vi "Car_Wash.vi"() -> ()   [LabVIEW 2021]
doc: "This is the car wash vi which simulates the car washing machine."
uses:
  Control/Queue_Operation_Select.ctl
  Control/Car_Wash_Data.ctl
  Control/Stage_Data.ctl
  Control/Timer_Operation_Select.ctl
  Control/Car_Wash_Indicators.ctl
  Control/INI_Operation_Select.ctl
  Control/Purchase_Selection.ctl
  Control/Car_Wash_Simulation_Switches.ctl
panel:
  out "Time":dbl format="%#_3g"
  out "Car_Wash_Indicators":T1 caption="Car Wash Indicators"
  in  "Stop":bool
  in  "Car_Wash_Simulation_Switches":T2 caption="Car Wash Simulation Switches"
  in  "Purchase_Selection":T3 caption="Purchase Selection"
  out "Error_Out":errorcluster
  in  "Error_In":errorcluster
  # "Sec"
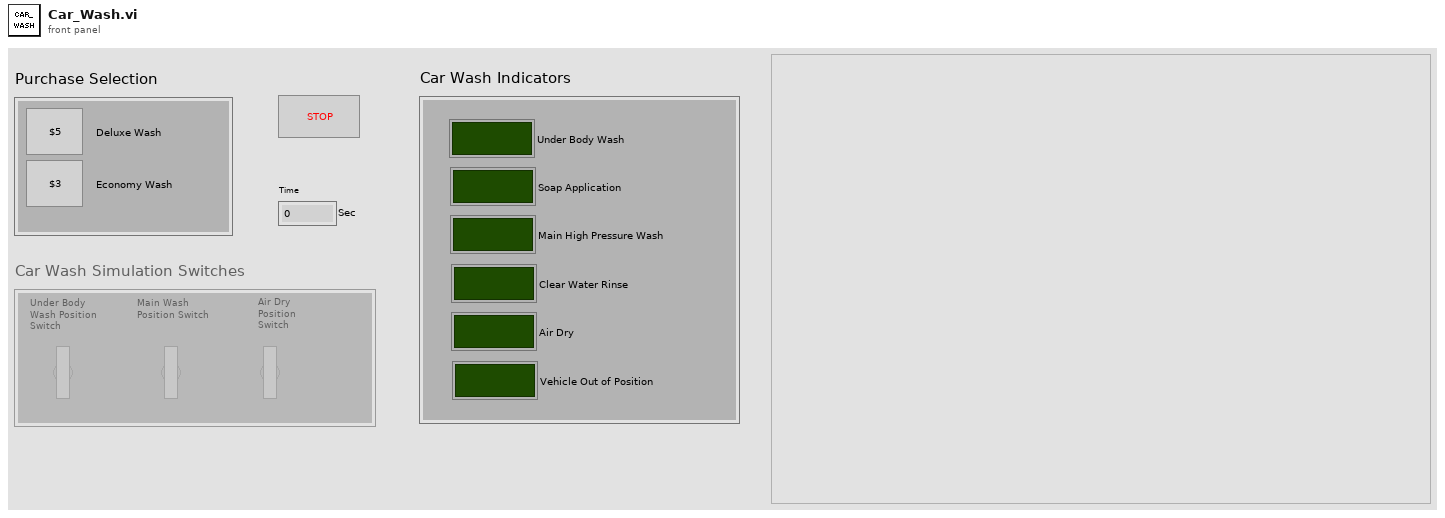
[diagram p1: front panel]
types:
  T1 = typedef "Car_Wash_Indicators.ctl" = cluster{"Under_Body_Wash":bool, "Soap_Application":bool, "Main_High_Pressure_Wash":bool, "Clear_Water_Rinse":bool, "Air_Dry":bool, "Vehicle_Out_of_Position":bool}
  T2 = typedef "Car_Wash_Simulation_Switches.ctl" = cluster{"Under_Body_Wash":bool, "Main_Wash":bool, "Dry_Wash":bool}
  T3 = typedef "Purchase_Selection.ctl" = cluster{"Deluxe_Wash":bool, "Economy_Wash":bool}
  T4 = typedef "Queue_Operation_Select.ctl" = enum16{"Obtain_Queue", "Enqueue", "Enqueue_N", "Enqueue_at_First", "Dequeue", "Flush_Queue", "Release_Queue"}
  T5 = typedef "Timer_Operation_Select.ctl" = enum16{"Start_Timer", "Pause_Timer", "Time_Out?", "Stop_Timer"}
  T6 = typedef "Car_Wash_Data.ctl" = cluster{"Car_Wash_Indicator_F":bool[], "Vehicle_Out_of_Position_F":bool, "Stage_1_Process_Data":T7[], "Stage_2_Process_Data":T7[], "Stage_3_Process_Data":T7[], "Stage_1_Process":i32, "Stage_2_Process":i32, "Stage_3_Process":i32, "Stage_1_Process_Started?":bool, "Stage_2_Process_Started?":bool, "Stage_3_Process_Started?":bool, "Current_Process_Stage":i32, "Enable_Control_Reference":refnum<vi>, "Disable_Control_Reference":refnum<vi>, "Car_Wash_Indicators":T1, "Latest_Car_Wash_Switch_Change":bool[], "Time":dbl}
  T7 = typedef "Stage_Data.ctl" = cluster{"Stage":i32, "Do?":bool, "Time_Required":i32}
  T8 = typedef "INI_Operation_Select.ctl" = enum16{"Read", "Write"}
  T9 = enum8{"Enabled", "Disabled", "Disabled and Grayed Out"}
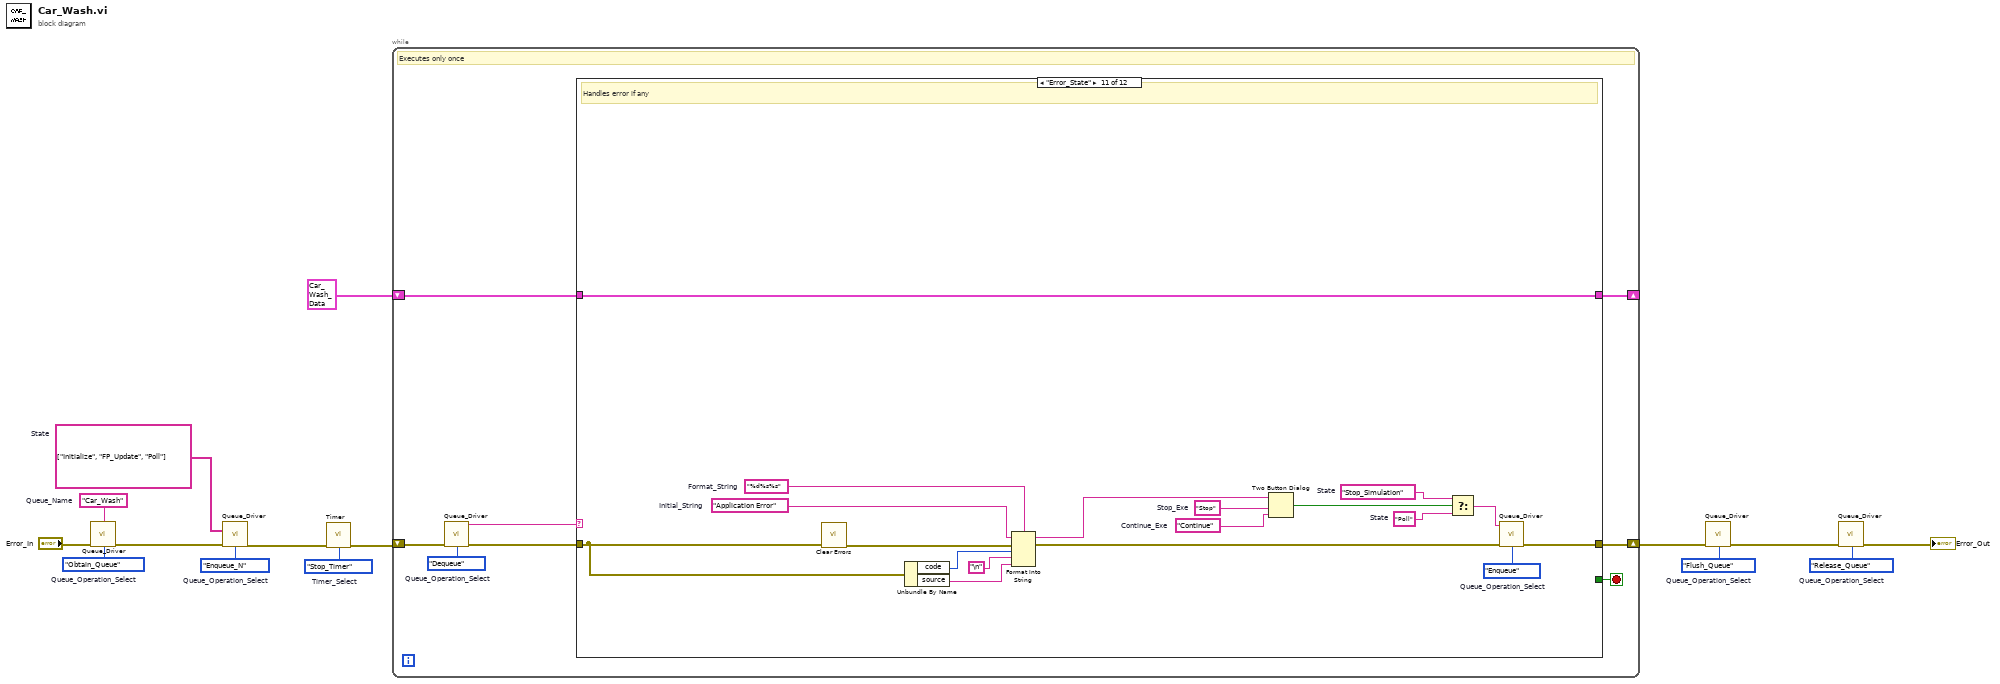
[diagram p0: block diagram]
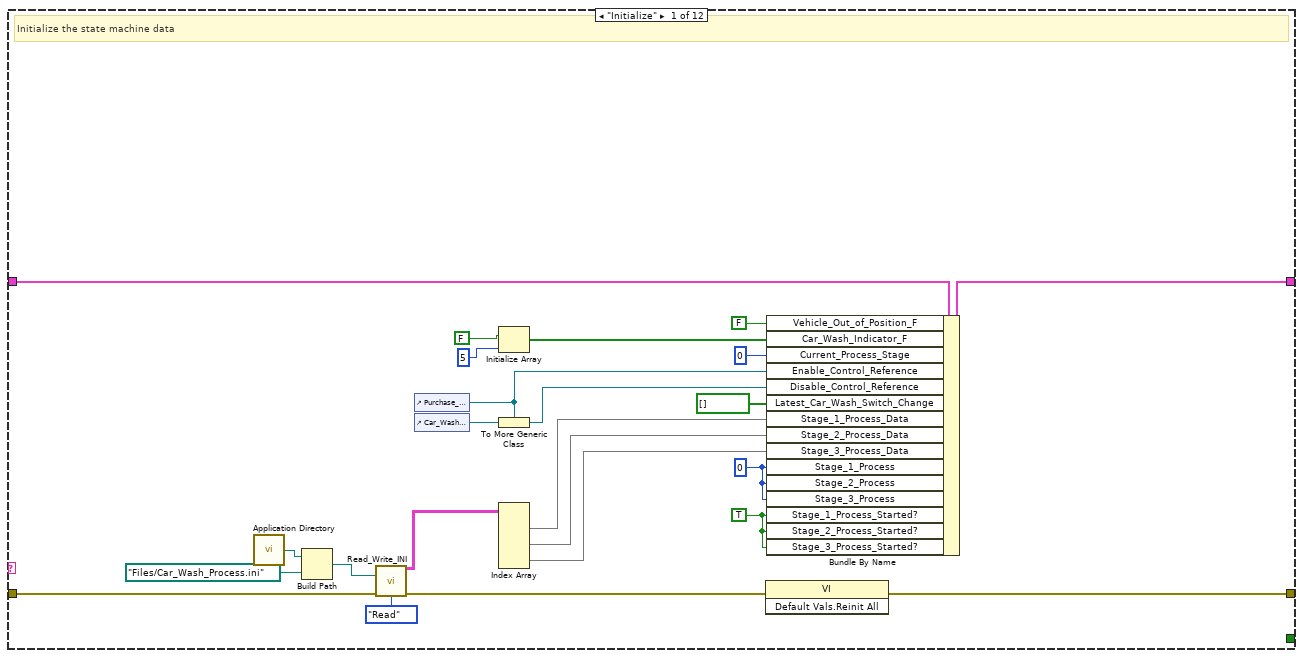
[diagram p2: hidden frame]
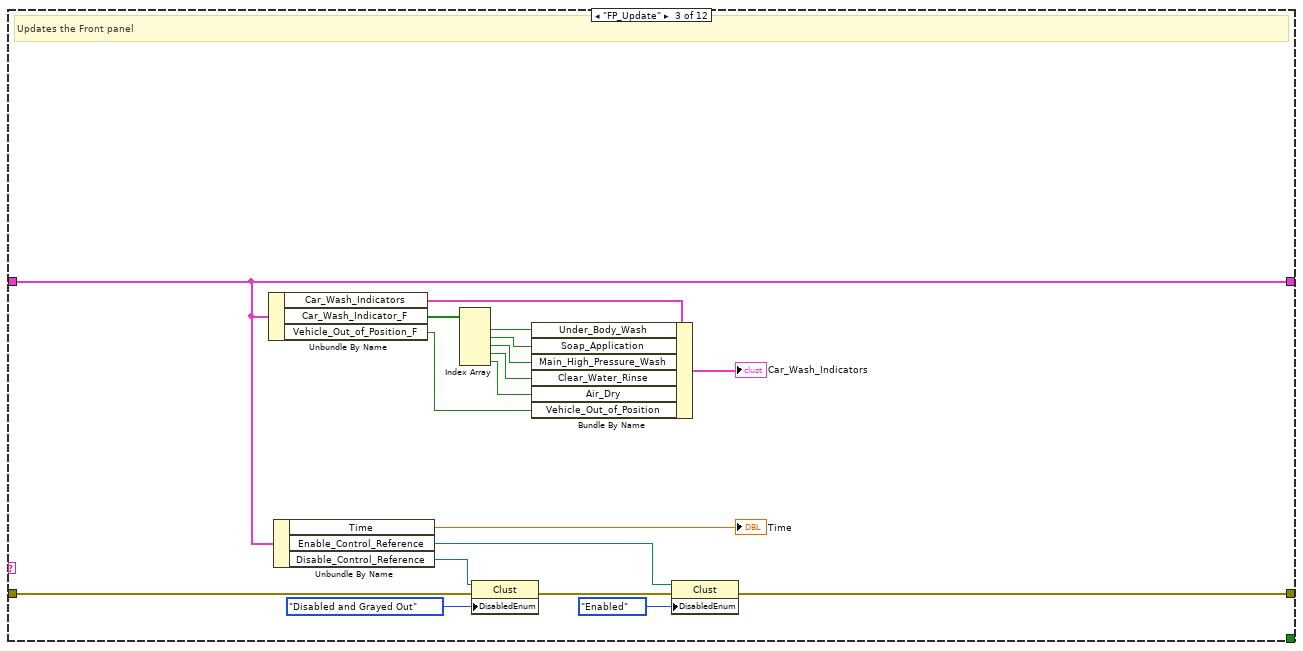
[diagram p4: hidden frame]
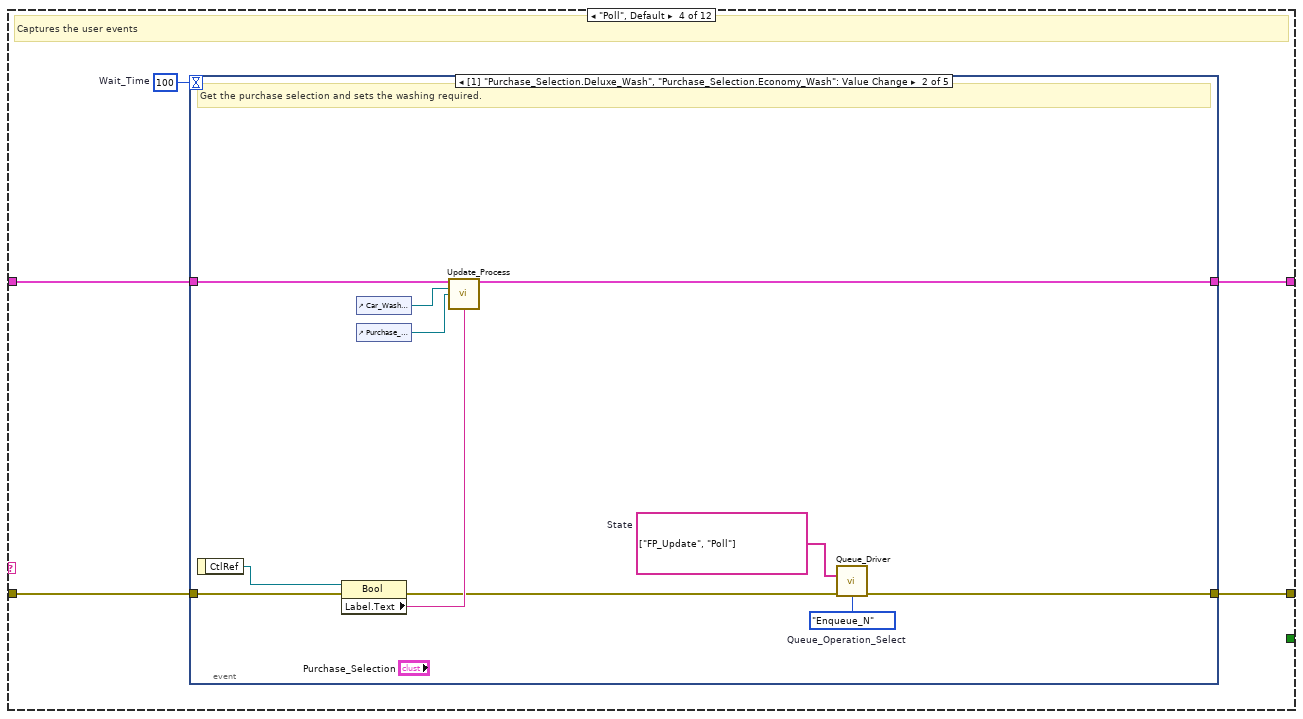
[diagram p5: hidden frame]
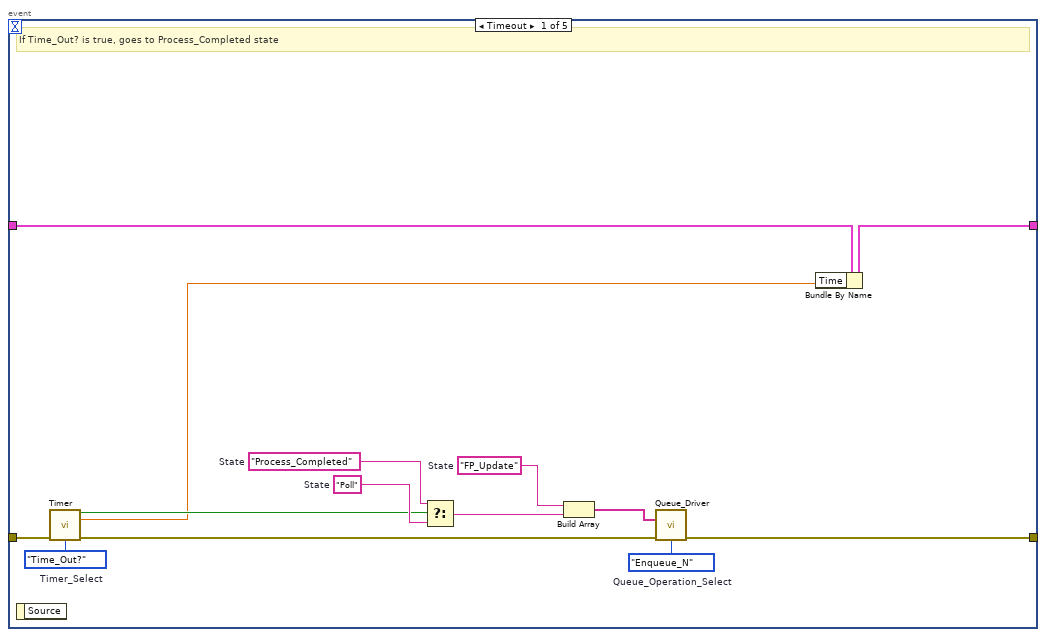
[diagram p6: hidden frame]
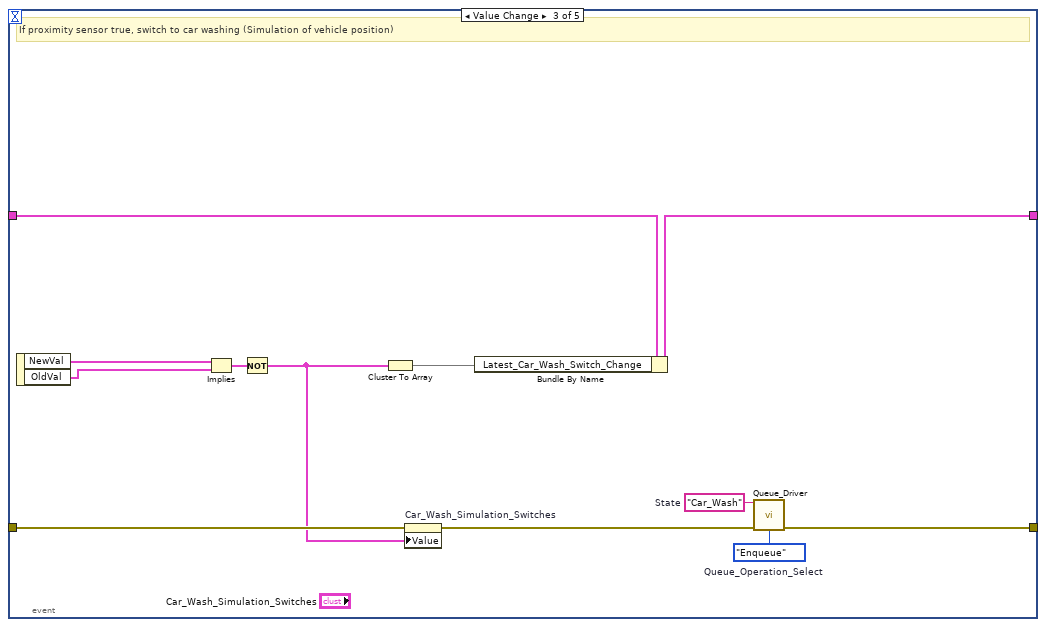
[diagram p7: hidden frame]
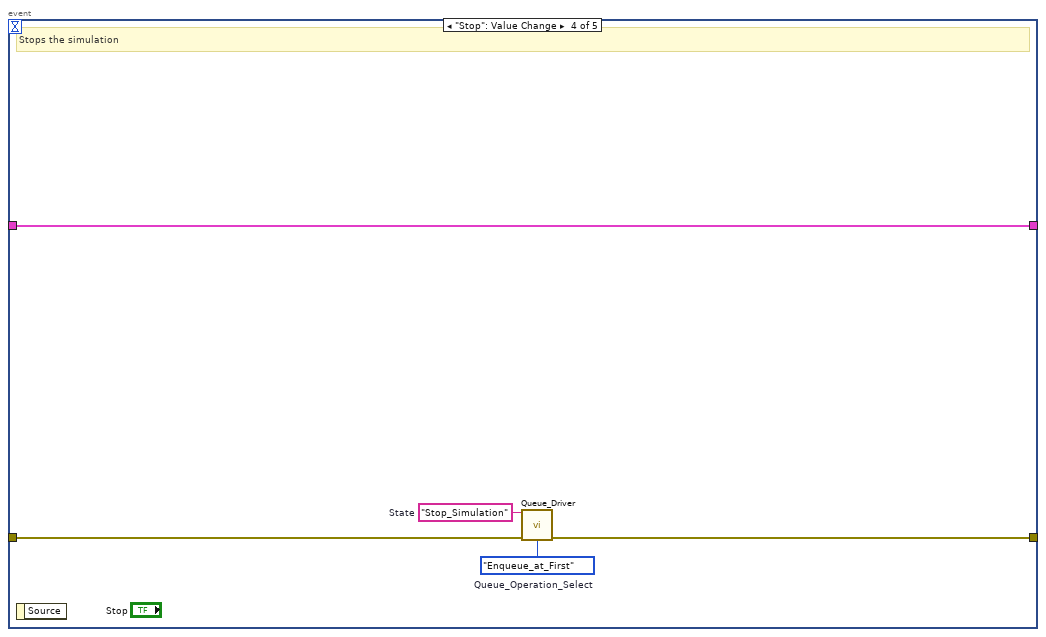
[diagram p8: hidden frame]
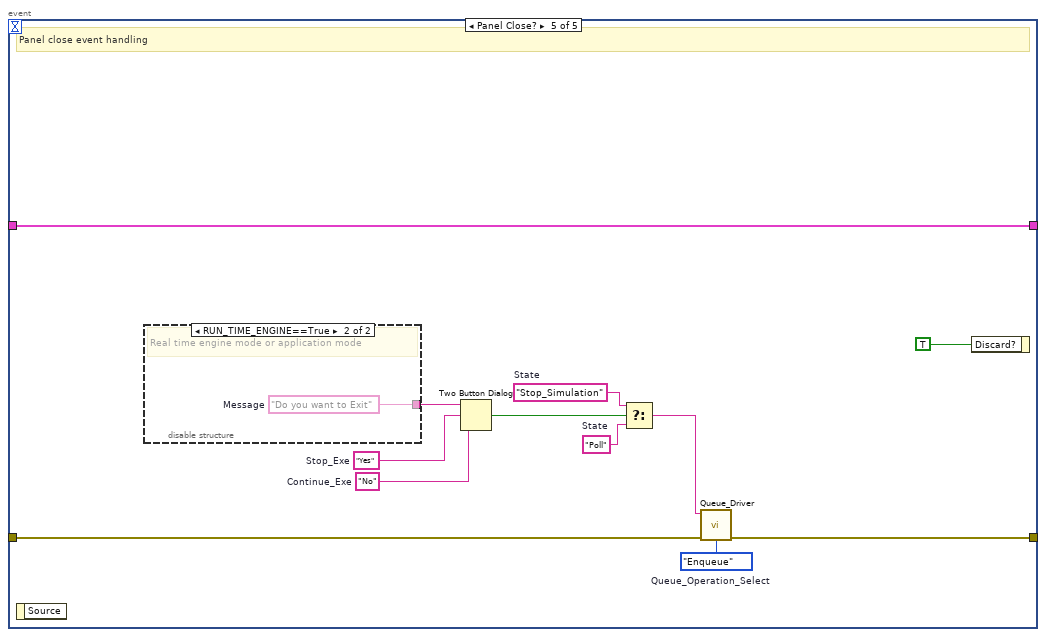
[diagram p9: hidden frame]
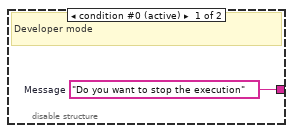
[diagram p10: hidden frame]
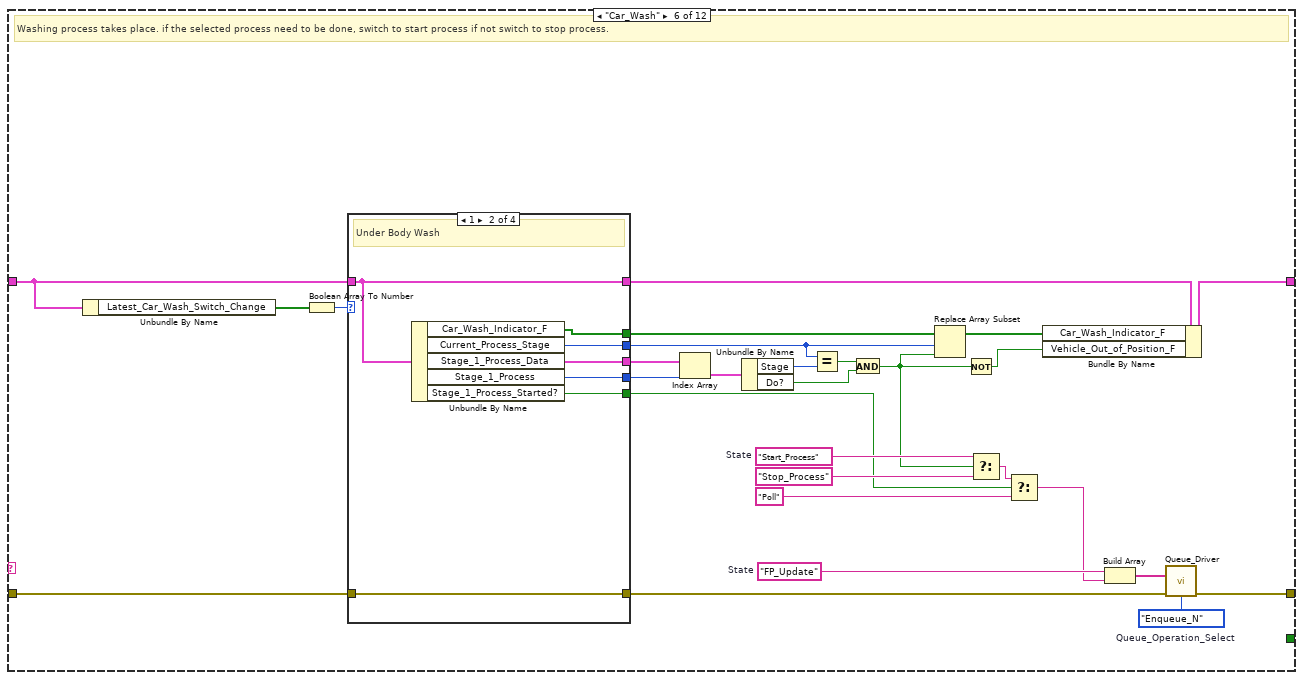
[diagram p12: hidden frame]
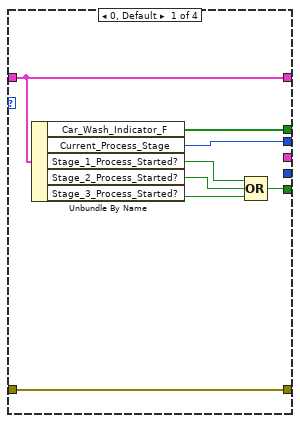
[diagram p13: hidden frame]
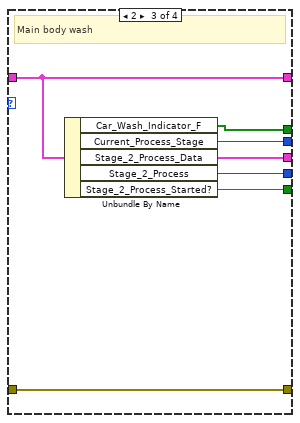
[diagram p14: hidden frame]
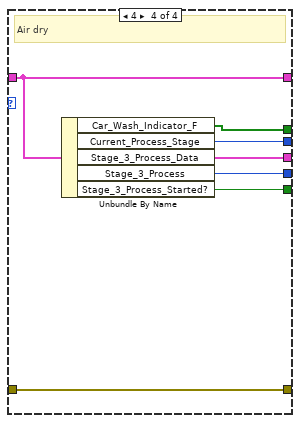
[diagram p15: hidden frame]
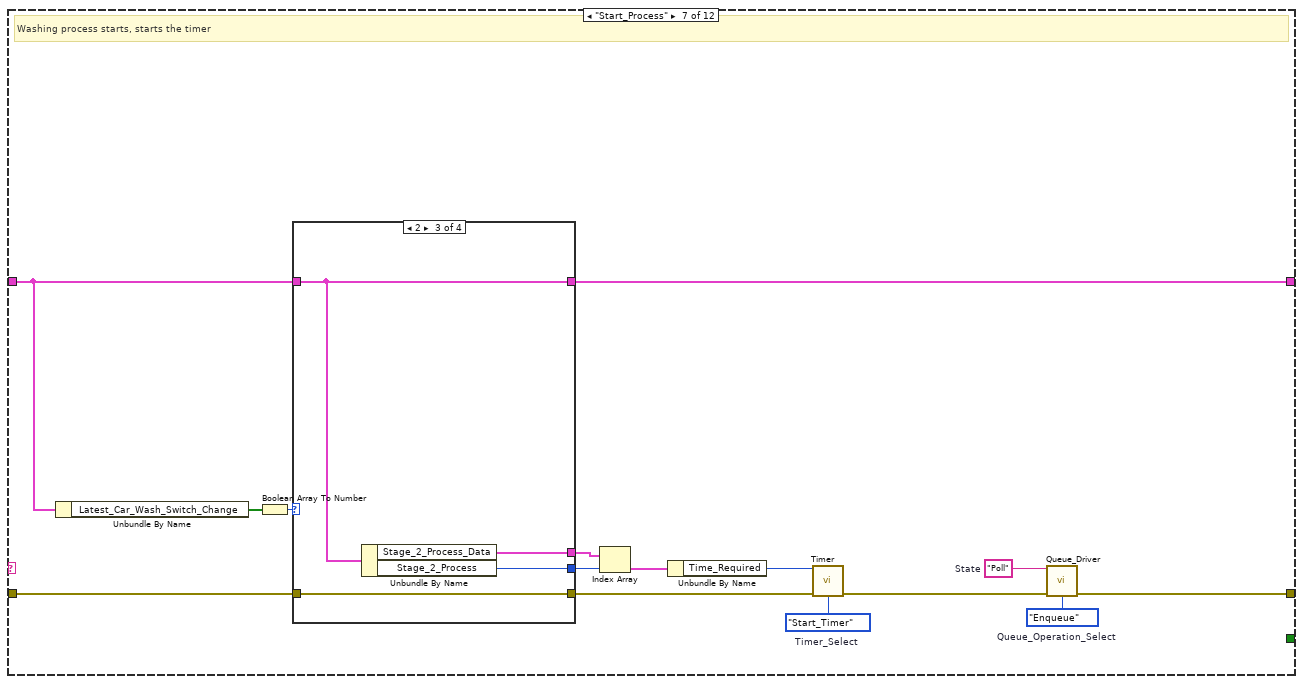
[diagram p16: hidden frame]
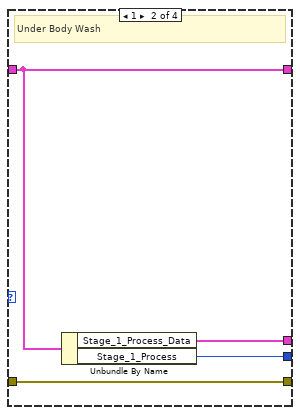
[diagram p18: hidden frame]
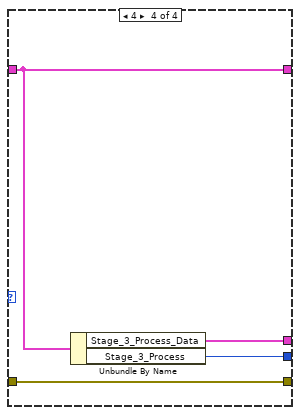
[diagram p19: hidden frame]
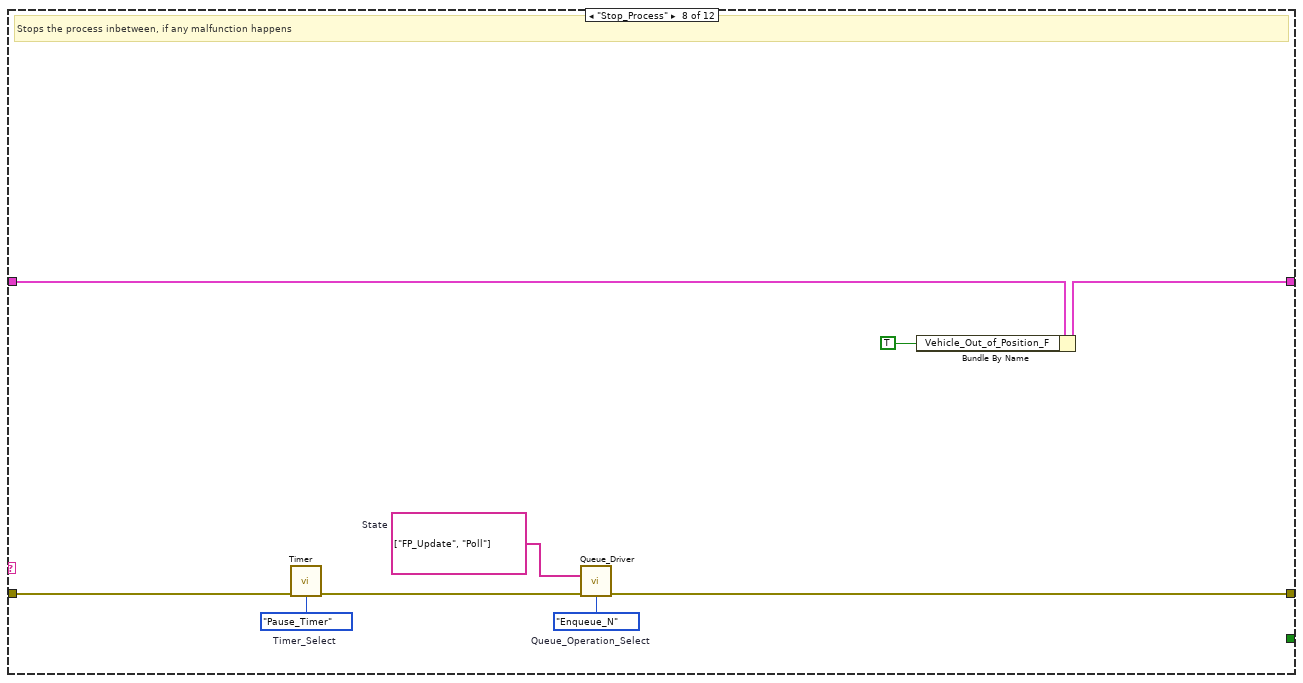
[diagram p20: hidden frame]
diagram:
  w2 = Queue_Operation_Select."Release_Queue"  # Queue_Operation_Select
  w4 = Queue_Operation_Select."Flush_Queue"  # Queue_Operation_Select
  w6 = Timer_Operation_Select."Stop_Timer"  # Timer_Select
  w9 = string[] ["Initialize", "FP_Update", "Poll"]  # State
  w10 = Queue_Operation_Select."Enqueue_N"  # Queue_Operation_Select
  w12 = "Car_Wash"  # Queue_Name
  w13 = Queue_Operation_Select."Obtain_Queue"  # Queue_Operation_Select
  n1 = call "Queue_Driver.vi"("Queue_Name"=w12, "Error_In"="Error_In", "Queue_Operation_Select"=w13) -> ("Error_Out"=w14:errorcluster)  [unwired: 11 in, 1 out]
  n2 = call "Queue_Driver.vi"("Data_In_N"=w9, "Error_In"=w14, "Queue_Operation_Select"=w10) -> ("Error_Out"=w11:errorcluster)  [unwired: 11 in, 1 out]
  n3 = call "Timer.vi"("Error_In"=w11, "Timer_Select"=w6) -> ("Error_Out"=w7:errorcluster)  [unwired: 11 in, 2 out]
  n4 = while {
    shift-right: [w18] -> _
    shift-left: T6 {"Car_Wash_Indicator_F"=[], "Vehicle_Out_of_Position_F"=FALSE, "Stage_1_Process_Data"=[], "Stage_2_Process_Data"=[], "Stage_3_Process_Data"=[], "Stage_1_Process"=0, "Stage_2_Process"=0, "Stage_3_Process"=0, "Stage_1_Process_Started?"=FALSE, "Stage_2_Process_Started?"=FALSE, "Stage_3_Process_Started?"=FALSE, "Current_Process_Stage"=0, "Enable_Control_Reference"=refnum, "Disable_Control_Reference"=refnum, "Car_Wash_Indicators"={"Under_Body_Wash"=FALSE, "Soap_Application"=FALSE, "Main_High_Pressure_Wash"=FALSE, "Clear_Water_Rinse"=FALSE, "Air_Dry"=FALSE, "Vehicle_Out_of_Position"=FALSE}, "Latest_Car_Wash_Switch_Change"=[], "Time"=0.0} -> [w19]
    shift-right: [w16] -> w1
    shift-left: w7 -> [w23]
    stop <- w17 stop-if-true
    w20 = Queue_Operation_Select."Dequeue"  # Queue_Operation_Select
    # "Executes only once"
    n5 = call "Queue_Driver.vi"("Error_In"=w23, "Queue_Operation_Select"=w20) -> ("Data_Out"=w21:string, "Error_Out"=w22:errorcluster)  [unwired: 12 in]
    n6 = case shown="\"Error_State\"" w21 {
      tunnel: w22 -> [w28 w49 w53 w68 w130 w149 w198 w225 w231 w255 w264 w277]
      tunnel: [w29 w49 w52 w72 w130 w158 w190 w224 w229 w255 w261 w274] -> w16
      tunnel: w19 -> [w47 w48 w51 w71 w129 w152 w199 w219 w237 w254 w273 w276]
      tunnel: [w46 w48 w51 w70 w129 w154 w191 w218 w234 w254 w273 w276] -> w18
      tunnel: [_ _ _ _ _ _ _ _ _ _ _ TRUE] -> w17
      frame "Initialize" {
        w38 = TRUE ("Process_Started?")
        w41 = 0 ("Stage_1_Process")
        # "Initialize the state machine data"
        n7 = call <vilib>:"Application Directory.vi"() -> ("Application Directory"=w34:path)
        n8 = Build Path(base path=w34, name or relative path=path "Files/Car_Wash_Process.ini") -> (appended path=w26:path)
        n9 = call "Read_Write_INI.vi"("File_Path"=w26, "Error_In"=w28, "INI_Select"=INI_Operation_Select."Read") -> ("Process_Data_Out"=w25:T7[][], "Error_Out"=w27:errorcluster)  [unwired: 11 in]
        n10 = control-ref of="Purchase_Selection"() -> (w42:refnum<vi>)
        n11 = control-ref of="Car_Wash_Simulation_Switches"() -> (w44:refnum<vi>)
        n12 = Initialize Array(FALSE ("Boolean"), 5 ("dimension size")) -> (w32:bool[])
        n13 = To More Generic Class(target class=w42, reference=w44) -> (generic class reference=w43:refnum<vi>)
        n14 = Index Array(array=w25) -> (element #1=w37:T7[], element #2=w36:T7[], element #3=w35:T7[])  [unwired: 6 in]
        n15 = invoke class="VI" method="Default Vals.Reinit All"(error in=w27) -> (error out=w29:errorcluster)  [unwired: 2 in, 2 out]
        n16 = Bundle By Name(cluster=w47, "Vehicle_Out_of_Position_F"=FALSE, "Car_Wash_Indicator_F"=w32, "Current_Process_Stage"=0, "Enable_Control_Reference"=w42, "Disable_Control_Reference"=w43, "Latest_Car_Wash_Switch_Change"=bool[] [], "Stage_1_Process_Data"=w37, "Stage_2_Process_Data"=w36, "Stage_3_Process_Data"=w35, "Stage_1_Process"=w41, "Stage_2_Process"=w41, "Stage_3_Process"=w41, "Stage_1_Process_Started?"=w38, "Stage_2_Process_Started?"=w38, "Stage_3_Process_Started?"=w38) -> (w46:T6)
      }
      frame "-----User_Update_States-----" {
        # "States after this are user update states"
      }
      frame "FP_Update" {
        # "Updates the Front panel"
        n17 = Unbundle By Name(w51) -> ("Car_Wash_Indicators"=w67:T1, "Car_Wash_Indicator_F"=w65:bool[], "Vehicle_Out_of_Position_F"=w64:bool)
        n18 = Unbundle By Name(w51) -> ("Time"=→"Time":dbl, "Enable_Control_Reference"=w57:refnum<vi>, "Disable_Control_Reference"=w56:refnum<vi>)
        n19 = Index Array(array=w65) -> (element #1=w63:bool, element #2=w62:bool, element #3=w61:bool, element #4=w60:bool, element #5=w59:bool)  [unwired: 5 in]
        n20 = property on="Property Node" class="Clust"(reference=w56, error in=w53, "DisabledEnum"=T9."Disabled and Grayed Out" ("Disabled")) -> (error out=w58:errorcluster)  [unwired: 1 out]
        n21 = Bundle By Name(cluster=w67, "Under_Body_Wash"=w63, "Soap_Application"=w62, "Main_High_Pressure_Wash"=w61, "Clear_Water_Rinse"=w60, "Air_Dry"=w59, "Vehicle_Out_of_Position"=w64) -> (→"Car_Wash_Indicators":T1)
        n22 = property on="Property Node" class="Clust"(reference=w57, error in=w58, "DisabledEnum"=T9."Enabled" ("Disabled")) -> (error out=w52:errorcluster)  [unwired: 1 out]
      }
      frame "Poll", Default {
        w69 = 100  # Wait_Time
        # "Captures the user events"
        n23 = event shown="[1] \"Purchase_Selection.Deluxe_Wash\", \"Purchase_Selection.Economy_Wash\": Value Change" {
          selector: _ -> [_ _ _ _ _]
          dyn-events: _ -> [_ _ _ _ _]
          timeout: w69 -> [_ _ _ _ _]
          tunnel: [w84 w92 w100 w113 w125] -> w72
          tunnel: w71 -> [w76 w96 w108 w114 w126]
          tunnel: [w75 w95 w107 w114 w126] -> w70
          tunnel: w68 -> [w73 w89 w105 w110 w115]
          event Timeout {
            w78 = "FP_Update"  # State
            w81 = "Poll"  # State
            w82 = "Process_Completed"  # State
            w83 = Queue_Operation_Select."Enqueue_N"  # Queue_Operation_Select
            w85 = Timer_Operation_Select."Time_Out?"  # Timer_Select
            # "If Time_Out? is true, goes to Process_Completed state"
            n24 = event-data() -> ()  [unwired: 1 in, 1 out]
            n25 = call "Timer.vi"("Error_In"=w73, "Timer_Select"=w85) -> ("Time_Out?"=w80:bool, "Time"=w74:dbl, "Error_Out"=w86:errorcluster)  [unwired: 11 in]
            n26 = Select(t=w82, s=w80, f=w81) -> (s? t:f=w79:string)
            n27 = Build Array(w78, w79) -> (w77:string[])
            n28 = call "Queue_Driver.vi"("Data_In_N"=w77, "Error_In"=w86, "Queue_Operation_Select"=w83) -> ("Error_Out"=w84:errorcluster)  [unwired: 11 in, 1 out]
            n29 = Bundle By Name(cluster=w76, "Time"=w74) -> (w75:T6)
          }
          event Value Change {
            w90 = string[] ["FP_Update", "Poll"]  # State
            w91 = Queue_Operation_Select."Enqueue_N"  # Queue_Operation_Select
            # "Get the purchase selection and sets the washing required."
            n30 = event-data() -> ("CtlRef"=w97:refnum<vi>)  [unwired: 1 in]
            n31 = property on="Property Node" class="Bool"(reference=w97, error in=w89) -> (error out=w93:errorcluster, "Label.Text"=w94:string)  [unwired: 1 out]
            n32 = control-ref of="Car_Wash_Simulation_Switches"() -> (w88:refnum<vi>)
            n33 = control-ref of="Purchase_Selection"() -> (w87:refnum<vi>)
            n34 = call "Update_Process.vi"("Car_Wash_Data_In"=w96, "Car_Wash_Switch_Reference"=w88, "Purchase_Selection_Reference"=w87, "Label.Text"=w94) -> ("Car_Wash_Data_Out"=w95:T6)  [unwired: 11 in]
            n35 = call "Queue_Driver.vi"("Data_In_N"=w90, "Error_In"=w93, "Queue_Operation_Select"=w91) -> ("Error_Out"=w92:errorcluster)  [unwired: 11 in, 1 out]
          }
          event Value Change {
            w106 = "Car_Wash"  # State
            w109 = Queue_Operation_Select."Enqueue"  # Queue_Operation_Select
            # "If proximity sensor true, switch to car washing (Simulation of vehicle position)"
            n36 = event-data() -> ("NewVal"=w103:T2, "OldVal"=w101:T2)  [unwired: 1 in]
            n37 = Implies(1:w101, 2:w103) -> (0:w102:T2)
            n38 = Not(x=w102) -> (.not. x?=w98:T2)
            n39 = Cluster To Array(cluster=w98) -> (array=w104:bool[])
            n40 = property on="Car_Wash_Simulation_Switches" class="Clust (strict)"(error in=w105, "Value"=w98) -> (error out=w99:errorcluster)  [unwired: 1 in, 1 out]
            n41 = Bundle By Name(cluster=w108, "Latest_Car_Wash_Switch_Change"=w104) -> (w107:T6)
            n42 = call "Queue_Driver.vi"("Data_In"=w106, "Error_In"=w99, "Queue_Operation_Select"=w109) -> ("Error_Out"=w100:errorcluster)  [unwired: 11 in, 1 out]
          }
          event "Stop": Value Change {
            w111 = "Stop_Simulation"  # State
            w112 = Queue_Operation_Select."Enqueue_at_First"  # Queue_Operation_Select
            # "Stops the simulation"
            n43 = event-data() -> ()  [unwired: 1 in, 1 out]
            n44 = call "Queue_Driver.vi"("Data_In"=w111, "Error_In"=w110, "Queue_Operation_Select"=w112) -> ("Error_Out"=w113:errorcluster)  [unwired: 11 in, 1 out]
          }
          event Panel Close? {
            w118 = "No"  # Continue_Exe
            w117 = "Yes"  # Stop_Exe
            w121 = Queue_Operation_Select."Enqueue"  # Queue_Operation_Select
            w124 = "Stop_Simulation"  # State
            w123 = "Poll"  # State
            # "Panel close event handling"
            n45 = event-data() -> ()  [unwired: 1 in, 1 out]
            n46 = disable-structure "Conditional Disable Structure" shown="RUN_TIME_ENGINE==True" {
              disable-tunnel: [w127 w128] -> w116
              frame condition #0 (active) {
                w127 = "Do you want to stop the execution"  # Message
                # "Developer mode"
              }
              frame condition #1 {
                w128 = "Do you want to Exit"  # Message
                # "Real time engine mode or application mode"
              }
            }
            n47 = Two Button Dialog(message=w116, 1:w118, 2:w117) -> (T button?=w120:bool)
            n48 = Select(t=w124, s=w120, f=w123) -> (s? t:f=w122:string)
            n49 = call "Queue_Driver.vi"("Data_In"=w122, "Error_In"=w115, "Queue_Operation_Select"=w121) -> ("Error_Out"=w125:errorcluster)  [unwired: 11 in, 1 out]
            n50 = event-data ("Event Filter Node")("Discard?"=TRUE) -> ()  [unwired: 1 in, 1 out]
          }
        }
      }
      frame "-------Washing_States-------" {
        # "States after this are Wasing process states"
      }
      frame "Car_Wash" {
        w141 = "FP_Update"  # State
        w155 = "Start_Process"  # State
        w157 = Queue_Operation_Select."Enqueue_N"  # Queue_Operation_Select
        # "Washing process takes place. if the selected process need to be done, switch to start process if not switch to stop process."
        n51 = Unbundle By Name(w152) -> ("Latest_Car_Wash_Switch_Change"=w146:bool[])
        n52 = Boolean Array To Number(Boolean array=w146) -> (number=w140:u32)
        n53 = case shown="1" w140 {
          tunnel: w152 -> [w165 w173 w179 w182]
          tunnel: [w165 w173 w179 w182] -> w151
          tunnel: [w166 w172 w180 w187] -> w150
          tunnel: w149 -> [w166 w172 w180 w187]
          tunnel: [_ w171 w177 w184] -> w148
          tunnel: [_ w170 w175 w183] -> w147
          tunnel: [w164 w169 w178 w186] -> w144
          tunnel: [w159 w168 w176 w185] -> w143
          tunnel: [w161 w167 w174 w181] -> w135
          frame 0, Default {
            n54 = Unbundle By Name(w165) -> ("Car_Wash_Indicator_F"=w164:bool[], "Current_Process_Stage"=w159:i32, "Stage_1_Process_Started?"=w160:bool, "Stage_2_Process_Started?"=w163:bool, "Stage_3_Process_Started?"=w162:bool)
            n55 = Compound Arithmetic op=OR(w160, w163, w162) -> (w161:bool)
          }
          frame 1 {
            # "Under Body Wash"
            n56 = Unbundle By Name(w173) -> ("Car_Wash_Indicator_F"=w169:bool[], "Current_Process_Stage"=w168:i32, "Stage_1_Process_Data"=w171:T7[], "Stage_1_Process"=w170:i32, "Stage_1_Process_Started?"=w167:bool)
          }
          frame 2 {
            # "Main body wash"
            n57 = Unbundle By Name(w179) -> ("Car_Wash_Indicator_F"=w178:bool[], "Current_Process_Stage"=w176:i32, "Stage_2_Process_Data"=w177:T7[], "Stage_2_Process"=w175:i32, "Stage_2_Process_Started?"=w174:bool)
          }
          frame 4 {
            # "Air dry"
            n58 = Unbundle By Name(w182) -> ("Car_Wash_Indicator_F"=w186:bool[], "Current_Process_Stage"=w185:i32, "Stage_3_Process_Data"=w184:T7[], "Stage_3_Process"=w183:i32, "Stage_3_Process_Started?"=w181:bool)
          }
        }
        n59 = Index Array(array=w148, index=w147) -> (element=w156:T7)
        n60 = Unbundle By Name(w156) -> ("Stage"=w153:i32, "Do?"=w131:bool)
        n61 = Equal?(x=w143, y=w153) -> (x = y?=w134:bool)
        n62 = And(x=w134, y=w131) -> (x .and. y?=w132:bool)
        n63 = Replace Array Subset(array=w144, new element=w132, index=w143) -> (w145:bool[])
        n64 = Not(x=w132) -> (.not. x?=w133:bool)
        n65 = Select(t=w155, s=w132, f="Stop_Process") -> (s? t:f=w139:string)
        n66 = Select(t=w139, s=w135, f="Poll") -> (s? t:f=w138:string)
        n67 = Bundle By Name(cluster=w151, "Car_Wash_Indicator_F"=w145, "Vehicle_Out_of_Position_F"=w133) -> (w154:T6)
        n68 = Build Array(w141, w138) -> (w142:string[])
        n69 = call "Queue_Driver.vi"("Data_In_N"=w142, "Error_In"=w150, "Queue_Operation_Select"=w157) -> ("Error_Out"=w158:errorcluster)  [unwired: 11 in, 1 out]
      }
      frame "Start_Process" {
        w188 = "Poll"  # State
        w189 = Queue_Operation_Select."Enqueue"  # Queue_Operation_Select
        w201 = Timer_Operation_Select."Start_Timer"  # Timer_Select
        # "Washing process starts, starts the timer"
        n70 = Unbundle By Name(w199) -> ("Latest_Car_Wash_Switch_Change"=w196:bool[])
        n71 = Boolean Array To Number(Boolean array=w196) -> (number=w192:u32)
        n72 = case shown="2" w192 {
          tunnel: w199 -> [w204 w208 w211 w213]
          tunnel: [w204 w208 w211 w213] -> w191
          tunnel: [w203 w207 w212 w216] -> w197
          tunnel: w198 -> [w203 w207 w212 w216]
          tunnel: [_ w206 w210 w215] -> w195
          tunnel: [_ w205 w209 w214] -> w194
          frame 0, Default {
          }
          frame 1 {
            # "Under Body Wash"
            n73 = Unbundle By Name(w208) -> ("Stage_1_Process_Data"=w206:T7[], "Stage_1_Process"=w205:i32)
          }
          frame 2 {
            n74 = Unbundle By Name(w211) -> ("Stage_2_Process_Data"=w210:T7[], "Stage_2_Process"=w209:i32)
          }
          frame 4 {
            n75 = Unbundle By Name(w213) -> ("Stage_3_Process_Data"=w215:T7[], "Stage_3_Process"=w214:i32)
          }
        }
        n76 = Index Array(array=w195, index=w194) -> (element=w193:T7)
        n77 = Unbundle By Name(w193) -> ("Time_Required"=w200:i32)
        n78 = call "Timer.vi"("Wait_Time"=w200, "Error_In"=w197, "Timer_Select"=w201) -> ("Error_Out"=w202:errorcluster)  [unwired: 10 in, 2 out]
        n79 = call "Queue_Driver.vi"("Data_In"=w188, "Error_In"=w202, "Queue_Operation_Select"=w189) -> ("Error_Out"=w190:errorcluster)  [unwired: 11 in, 1 out]
      }
      frame "Stop_Process" {
        w220 = string[] ["FP_Update", "Poll"]  # State
        w221 = Timer_Operation_Select."Pause_Timer"  # Timer_Select
        w223 = Queue_Operation_Select."Enqueue_N"  # Queue_Operation_Select
        # "Stops the process inbetween, if any malfunction happens"
        n80 = call "Timer.vi"("Error_In"=w225, "Timer_Select"=w221) -> ("Error_Out"=w222:errorcluster)  [unwired: 11 in, 2 out]
        n81 = call "Queue_Driver.vi"("Data_In_N"=w220, "Error_In"=w222, "Queue_Operation_Select"=w223) -> ("Error_Out"=w224:errorcluster)  [unwired: 11 in, 1 out]
        n82 = Bundle By Name(cluster=w219, "Vehicle_Out_of_Position_F"=TRUE) -> (w218:T6)
      }
      frame "Process_Completed" {
        w226 = string[] ["Initialize", "Disable_Enable_Control", "FP_Update", "Poll"]  # State
        w227 = string[] ["FP_Update", "Car_Wash"]  # State
        w238 = Queue_Operation_Select."Enqueue_N"  # Queue_Operation_Select
        w239 = Timer_Operation_Select."Stop_Timer"  # Timer_Select
        # "If the washing process completed, move to next if any"
        n83 = Unbundle By Name(w237) -> ("Latest_Car_Wash_Switch_Change"=w236:bool[])
        n84 = Boolean Array To Number(Boolean array=w236) -> (number=w232:u32)
        n85 = case shown="Default" w232 {
          tunnel: w237 -> [w241 w244 w250 w252]
          tunnel: [w241 w243 w249 w253] -> w235
          tunnel: [w240 w242 w248 w251] -> w228
          tunnel: w227 -> [w240 w242 w246 _]
          tunnel: w226 -> [_ _ w245 w251]
          frame Default {
          }
          frame 1 {
            # "Under body wash"
            n86 = call "Under_Body_Wash.vi"("Car_Wash_Data_In"=w244) -> ("Car_Wash_Data_Out"=w243:T6)  [unwired: 14 in]
          }
          frame 2 {
            # "Main body wash"
            n87 = call "Main_Body_Wash.vi"("Car_Wash_Data_In"=w250) -> ("Car_Wash_Data_Out"=w249:T6, "Do?"=w247:bool)  [unwired: 13 in]
            n88 = Select(t=w245, s=w247, f=w246) -> (s? t:f=w248:string[])
          }
          frame 4 {
            # "Air dry"
            n89 = call "Air_Dry.vi"("Car_Wash_Data_In"=w252) -> ("Car_Wash_Data_Out"=w253:T6)  [unwired: 14 in]
          }
        }
        n90 = call "Timer.vi"("Error_In"=w231, "Timer_Select"=w239) -> ("Error_Out"=w230:errorcluster)  [unwired: 11 in, 2 out]
        n91 = Bundle By Name(cluster=w235, "Vehicle_Out_of_Position_F"=TRUE) -> (w234:T6)
        n92 = call "Queue_Driver.vi"("Data_In_N"=w228, "Error_In"=w230, "Queue_Operation_Select"=w238) -> ("Error_Out"=w229:errorcluster)  [unwired: 11 in, 1 out]
      }
      frame "---Exception_Handling_States---" {
        # "States after this Handles the exceptions."
      }
      frame "Error_State" {
        w257 = "Poll"  # State
        w258 = "Stop_Simulation"  # State
        w260 = Queue_Operation_Select."Enqueue"  # Queue_Operation_Select
        w269 = "%d%s%s"  # Format_String
        w270 = "Application Error"  # Initial_String
        w271 = "Stop"  # Stop_Exe
        w272 = "Continue"  # Continue_Exe
        # "Handles error if any"
        n93 = call <vilib>:"Clear Errors.vi"("error in (no error)"=w264) -> ("error out"=w267:errorcluster)  [unwired: 5 in, 1 out]
        n94 = Unbundle By Name(w264) -> ("code"=w266:i32, "source"=w265:string)
        n95 = Format Into String(format string=w269, initial string=w270, error in=w267, w266, "\n" ("Line Feed Constant"), w265) -> (resulting string=w262:string, error out=w263:errorcluster)
        n96 = Two Button Dialog(message=w262, 1:w272, 2:w271) -> (T button?=w259:bool)
        n97 = Select(t=w258, s=w259, f=w257) -> (s? t:f=w256:string)
        n98 = call "Queue_Driver.vi"("Data_In"=w256, "Error_In"=w263, "Queue_Operation_Select"=w260) -> ("Error_Out"=w261:errorcluster)  [unwired: 11 in, 1 out]
      }
      frame "Stop_Simulation" {
        # "Stops the simulation"
        n99 = disable-structure shown="RUN_TIME_ENGINE==True" {
          disable-tunnel: w277 -> [w279 w280]
          disable-tunnel: [w278 w280] -> w274
          frame condition #0 {
            n100 = invoke class="VI" method="FP.Close"(error in=w279) -> (error out=w278:errorcluster)  [unwired: 2 in, 2 out]
          }
          frame condition #1 (active) {
          }
        }
      }
    }
  }
  n101 = call "Queue_Driver.vi"("Error_In"=w1, "Queue_Operation_Select"=w4) -> ("Error_Out"=w5:errorcluster)  [unwired: 12 in, 1 out]
  n102 = call "Queue_Driver.vi"("Error_In"=w5, "Queue_Operation_Select"=w2) -> ("Error_Out"=→"Error_Out":errorcluster)  [unwired: 12 in, 1 out]
